vi "Count Objects Reduced.vi"(4 "State In":T1, 6 "Settings":T4={"Objects"=0, "Threshold"=128, "Reject Border"=FALSE, "Fill Holes"=FALSE, "Min Object Size"=FALSE, "Min Size"=3, "Max Object Size"=FALSE, "Max Size"=100, "Show Search Area"=FALSE, "Show Center"=TRUE, "Show Bounding Box"=TRUE} {"Objects" items=["Bright Objects", "Dark Objects"]; "Threshold" min=1 max=999999999 step=1; "Max Size" min=1 max=999999999 step=1; "Min Size" min=1 max=999999999 step=1}, 7 "Low/Tiny":bool, 8 "error in":errorcluster, 9 "Rectangle":T3 {"Rotation" min=-90.0 max=90.0 step=1.0 format="%.2f"; "Left" scale=0.0..1024.0; "Right" scale=0.0..1024.0}, 10 "Temp":T2, 11 "Image":T2) -> (0 "error out":errorcluster, 2 "Objects":T5[](array[typedef]) {"Aspect Ratio" format="%.2f"; "Orientation" format="%.2f"; "Area" format="%.2f"; "Object Center"."Y" format="%.2f"; "Object Center"."X" format="%.2f"}, 3 "Elapsed time (ms)":u32, 5 "Number of Objects":i32)   [LabVIEW 2015]
uses:
  TypeDefs Host/Object Info.ctl
  <vilib>/vision/Image Controls.llb/IMAQ Image.ctl
  TypeDefs Host/States.ctl
  <vilib>/vision/NI_Vision_Development_Module.lvlib
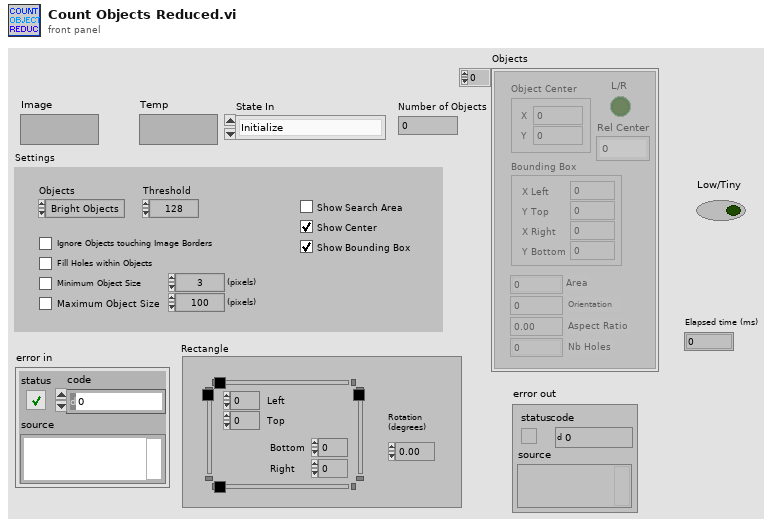
[diagram p1: front panel]
types:
  T1 = typedef "States.ctl" = enum16{"Initialize", "Calibrate", "Create", "Settings", "Shutdown"}
  T2 = typedef "IMAQ Image.ctl" = refnum<image>
  T3 = typedef "IMAQ Rectangle" = cluster{"Left":i32, "Top":i32, "Right":i32, "Bottom":i32, "Rotation":dbl}
  T4 = cluster{"Objects":u16, "Threshold":i32, "Reject Border":bool, "Fill Holes":bool, "Min Object Size":bool, "Min Size":i32, "Max Object Size":bool, "Max Size":i32, "Show Search Area":bool, "Show Center":bool, "Show Bounding Box":bool}
  T5 = typedef "Object Info.ctl" = cluster{"Object Center":cluster{"X":u16, "Y":u16}, "Bounding Box":cluster{"X Left":u16, "Y Top":u16, "X Right":u16, "Y Bottom":u16}, "Area":u16, "Orientation":u16, "Aspect Ratio":sgl, "Nb Holes":u16, "L/R":bool, "Rel Center":u16}
  T6 = typedef "Particle Parameters" = i32
  T7 = cluster{"Measurement Parameter":T6, "Range Lower Value":dbl, "Range Upper Value":dbl, "Range":bool, "Measurement Type":bool}[]
  T8 = typedef "ROI Descriptor" = cluster{"Global Rectangle":i32[], "Contours":cluster{"ID":enum32{"External", "Internal"}, "Type":u32, "Coordinates":i32[]}[]}
  T9 = cluster{"Measurement Parameter":T6, "Range Lower Value":dbl, "Range Upper Value":dbl, "Range":bool, "Measurement Type":bool}
  T10 = cluster{"Global Rectangle[0]":i32, "Global Rectangle[1]":i32}
  T11 = cluster{"[0]":u16, "[1]":u16, "[2]":u16, "[3]":u16, "[4]":u16, "[5]":u16, "[6]":u16, "[7]":u16, "[8]":u16, "[9]":u16, "[10]":u16}
  T12 = cluster{"[2]":u16, "[3]":u16, "[4]":u16, "[5]":u16}
  T13 = cluster{"X Left":u16, "Y Top":u16, "X Right":u16, "Y Bottom":u16}
  T14 = cluster{"Object Center":cluster{"X":u16, "Y":u16}, "Bounding Box":cluster{"X Left":u16, "Y Top":u16, "X Right":u16, "Y Bottom":u16}, "Area":u16, "Orientation":u16, "Aspect Ratio":sgl, "Nb Holes":u16}
  T15 = cluster{"Show Search Area":bool, "Show Center":bool, "Show Bounding Box":bool}
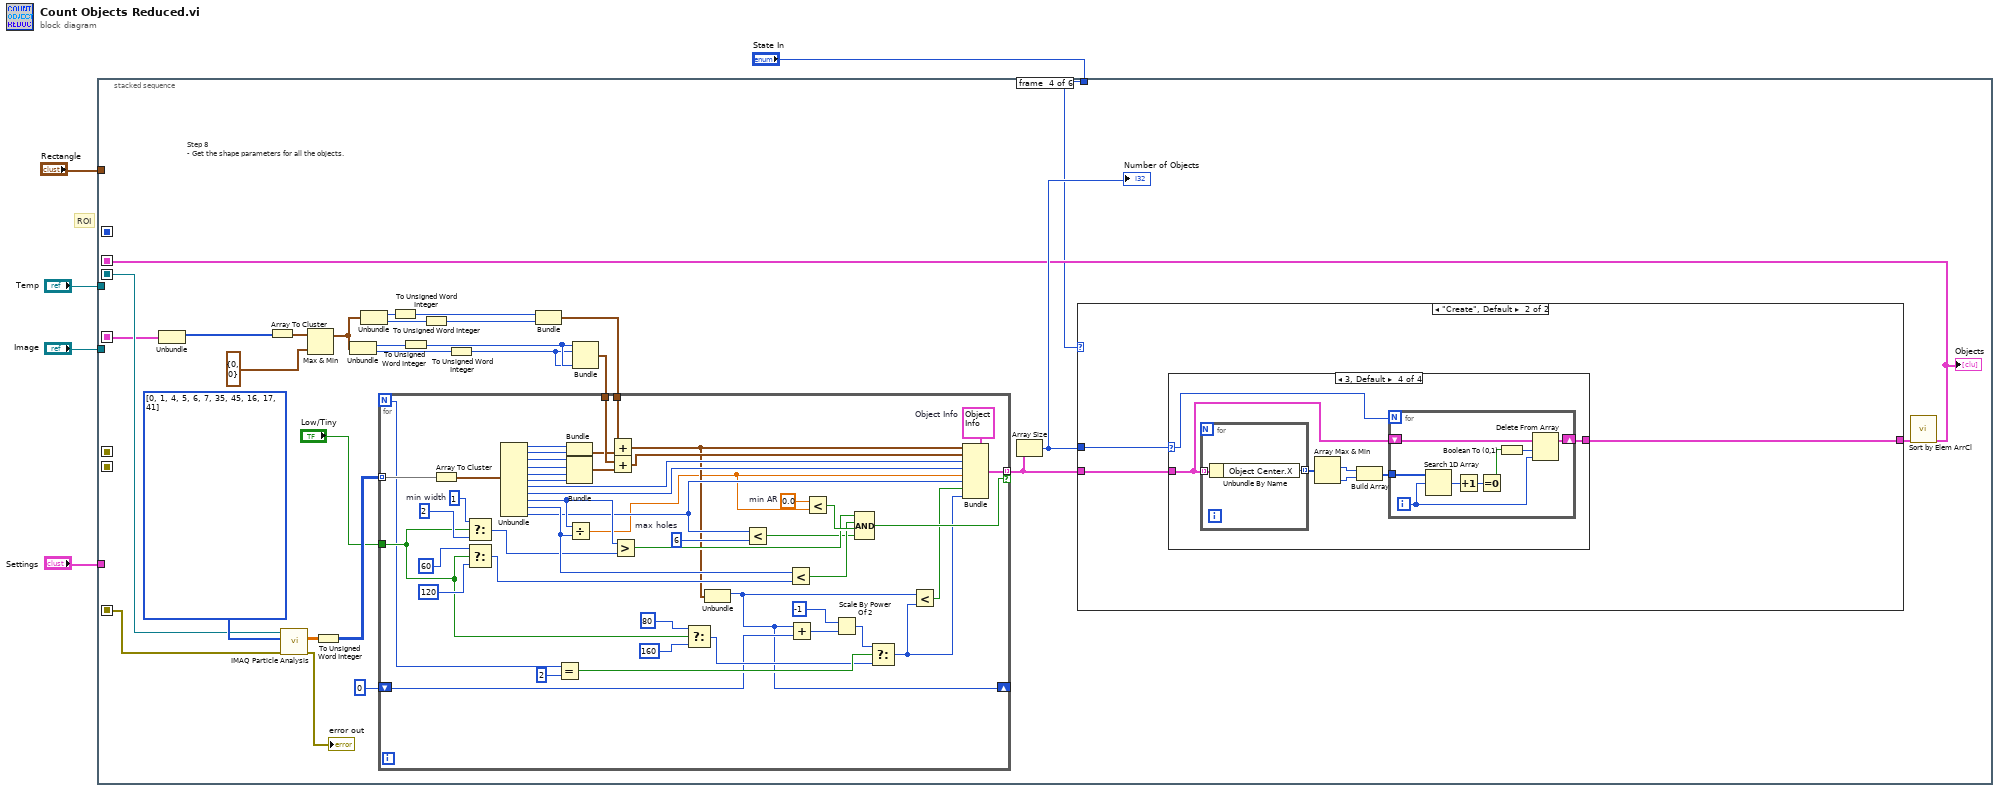
[diagram p0: block diagram]
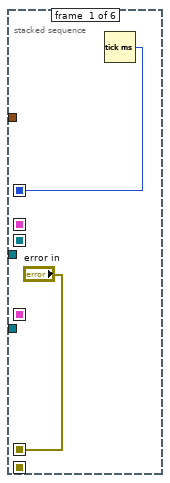
[diagram p2: hidden frame]
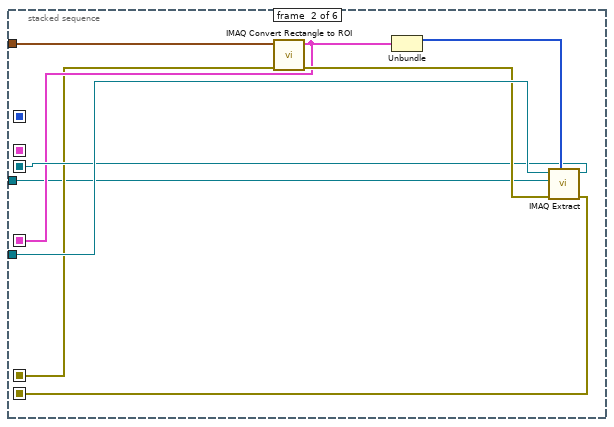
[diagram p3: hidden frame]
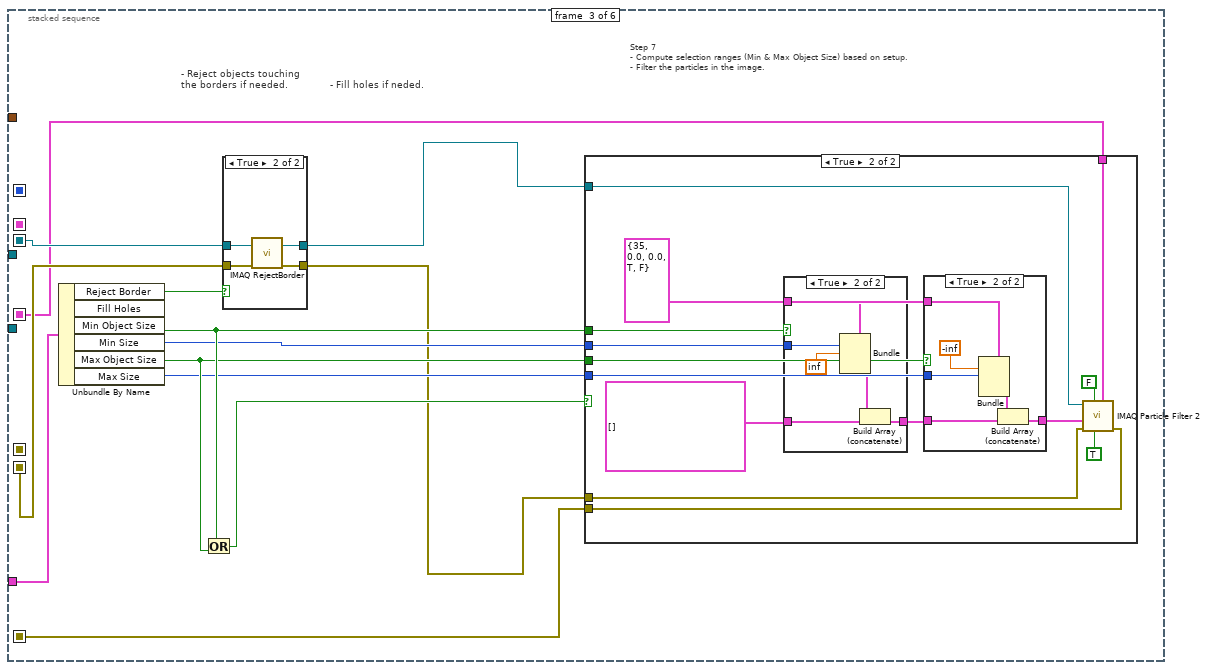
[diagram p4: hidden frame]
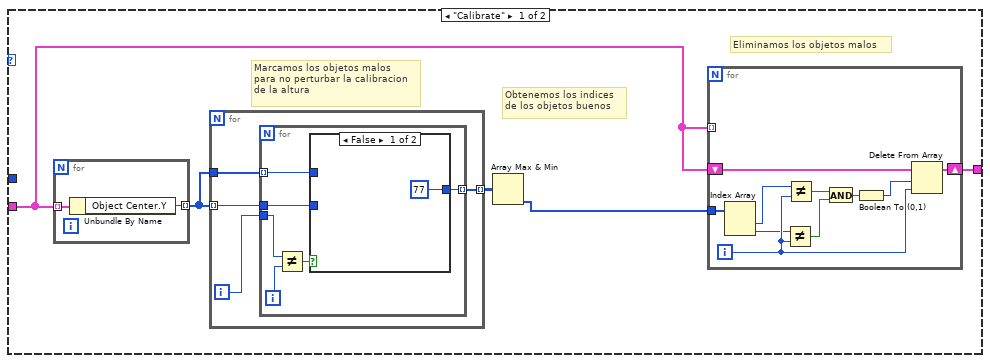
[diagram p9: hidden frame]
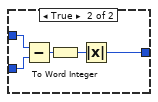
[diagram p10: hidden frame]
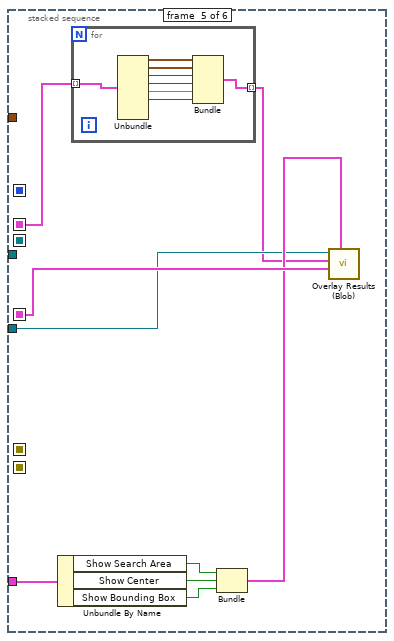
[diagram p14: hidden frame]
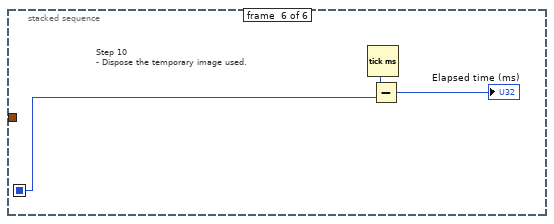
[diagram p15: hidden frame]
diagram:
  # "ROI"
  n1 = stacked-sequence {
    seq-local: [w7 _ _ _ _ _] -> [_ _ _ _ _ w217]
    seq-local: [_ _ _ w67 _ _] -> [_ _ _ _ w202 _]
    seq-local: [_ _ w23 _ _ _] -> [_ _ _ w82 _ _]
    seq-local: ["error in" _ _ _ _ _] -> [_ w9 _ _ _ _]
    seq-local: [_ w12 _ _ _ _] -> [_ _ w22 _ _ _]
    seq-local: [_ w11 _ _ _ _] -> [_ _ w21 w86 _ _]
    seq-local: [_ w10 _ _ _ _] -> [_ _ w19 w85 w201 _]
    tunnel: "Settings" -> [_ _ w28 _ w206 _]
    tunnel: "Image" -> [_ w16 _ _ w199 _]
    tunnel: "Rectangle" -> [_ w14 _ _ _ _]
    tunnel: "Temp" -> [_ w8 _ _ _ _]
    tunnel: "State In" -> [_ _ _ w66 _ _]
    frame #0 {
      n2 = Tick Count (ms)() -> (millisecond timer value=w7:u32)
    }
    frame #1 {
      n3 = call "IMAQ Convert Rectangle to ROI"("error in (no error)"=w9, "Rectangle"=w14) -> ("error out"=w13:errorcluster, "ROI Descriptor"=w10:T8)  [unwired: 7 out]
      n4 = Unbundle(w10) -> ("Global Rectangle"=w15:i32[])  [unwired: 1 out]
      n5 = call "IMAQ Extract"("Optional Rectangle"=w15, "error in (no error)"=w13, "Image Dst"=w8, "Image Src"=w16) -> ("error out"=w12:errorcluster, "Image Dst Out"=w11:T2)  [unwired: 2 in, 4 out]
    }
    frame #2 {
      # "- Fill holes if neded."
      # "- Reject objects touching the borders if needed."
      # "Step 7\n- Compute selection ranges (Min & Max Object Size) based on setup.\n- Filter the particles in the image."
      n6 = Unbundle By Name(w28) -> ("Reject Border"=w20:bool, "Min Object Size"=w27:bool, "Min Size"=w26:i32, "Max Object Size"=w25:bool, "Max Size"=w24:i32)  [unwired: 1 out]
      n7 = Or(x=w27, y=w25) -> (x .or. y?=w29:bool)
      n8 = case shown="True" w20 {
        tunnel: w21 -> [w31 w35]
        tunnel: w22 -> [w30 w34]
        tunnel: [w30 w32] -> w17
        tunnel: [w31 w33] -> w18
        frame False {
        }
        frame True {
          n9 = call "IMAQ RejectBorder"("error in (no error)"=w34, "Image Src"=w35) -> ("error out"=w32:errorcluster, "Image Dst Out"=w33:T2)  [unwired: 2 in, 2 out]
        }
      }
      n10 = case shown="True" w29 {
        tunnel: w27 -> [_ w50]
        tunnel: w26 -> [_ w49]
        tunnel: w25 -> [_ w48]
        tunnel: w24 -> [_ w47]
        tunnel: w17 -> [w36 w45]
        tunnel: [w36 w44] -> w23
        tunnel: w18 -> [_ w38]
        tunnel: w19 -> [_ w37]
        frame False {
        }
        frame True {
          w42 = T9 {"Measurement Parameter"=35, "Range Lower Value"=0.0, "Range Upper Value"=0.0, "Range"=TRUE, "Measurement Type"=FALSE} ("Selection Value")
          n11 = case shown="True" w50 {
            tunnel: T7 [] ("Selection Values") -> [w58 w64]
            tunnel: w49 -> [_ w61]
            tunnel: [w58 w62] -> w40
            tunnel: w42 -> [_ w59]
            frame False {
            }
            frame True {
              n12 = Bundle(cluster=w59, "Range Lower Value"=w61, "Range Upper Value"=inf) -> (w63:T9)  [unwired: 3 out]
              n13 = Build Array (concatenate)(w63, w64) -> (w62:T7)
            }
          }
          n14 = case shown="True" w48 {
            tunnel: w40 -> [w51 w57]
            tunnel: w47 -> [_ w54]
            tunnel: [w51 w55] -> w41
            tunnel: w42 -> [_ w52]
            frame False {
            }
            frame True {
              n15 = Bundle(cluster=w52, "Range Lower Value"=-inf, "Range Upper Value"=w54) -> (w56:T9)  [unwired: 3 out]
              n16 = Build Array (concatenate)(w56, w57) -> (w55:T7)
            }
          }
          n17 = call "IMAQ Particle Filter 2"("ROI Descriptor"=w37, "Keep/Remove Particles (F)"=TRUE ("Keep/Remove Particles"), "Connectivity 4/8 (8)"=FALSE ("Keep/Remove Particles"), "error in (no error)"=w45, "Selection Values"=w41, "Image Src"=w38) -> ("error out"=w44:errorcluster)  [unwired: 2 in, 3 out]
        }
      }
    }
    frame #3 {
      w87 = T6[] [0, 1, 4, 5, 6, 7, 35, 45, 16, 17, 41] items=["Center of Mass X", "Center of Mass Y", "First Pixel X", "First Pixel Y", "Bounding Rect Left", "Bounding Rect Top", "Bounding Rect Right", "Bounding Rect Bottom", "Max Feret Diameter Start X", "Max Feret Diameter Start Y", "Max Feret Diameter End X", "Max Feret Diameter End Y", "Max Horiz. Segment Length Left", "Max Horiz. Segment Length Right", "Max Horiz. Segment Length Row", "-", "Bounding Rect Width", "Bounding Rect Height", "Bounding Rect Diagonal", "Perimeter", "Convex Hull Perimeter", "Holes' Perimeter", "Max Feret Diameter", "Equivalent Ellipse Major Axis", "Equivalent Ellipse Minor Axis", "Equivalent Ellipse Minor Axis (Feret)", "Equivalent Rect Long Side", "Equivalent Rect Short Side", "Equivalent Rect Diagonal", "Equivalent Rect Short Side (Feret)", "Average Horiz. Segment Length", "Average Vert. Segment Length", "Hydraulic Radius", "Waddel Disk Diameter", "-", "Area", "Holes' Area", "Particle & Holes' Area", "Convex Hull Area", "Image Area", "-", "Number of Holes", "Number of Horiz. Segments", "Number of Vert. Segments", "-", "Orientation", "Max Feret Diameter Orientation", "-", "% Area/Image Area", "% Area/(Particle & Holes' Area)", "Ratio of Equivalent Ellipse Axes", "Ratio of Equivalent Rect Sides", "-", "Elongation Factor", "Compactness Factor", "Heywood Circularity Factor", "Type Factor", "-", "Sum X", "Sum Y", "Sum XX", "Sum XY", "Sum YY", "Sum XXX", "Sum XXY", "Sum XYY", "Sum YYY", "-", "Moment of Inertia XX", "Moment of Inertia XY", "Moment of Inertia YY", "Moment of Inertia XXX", "Moment of Inertia XXY", "Moment of Inertia XYY", "Moment of Inertia YYY", "Norm. Moment of Inertia XX", "Norm. Moment of Inertia XY", "Norm. Moment of Inertia YY", "Norm. Moment of Inertia XXX", "Norm. Moment of Inertia XXY", "Norm. Moment of Inertia XYY", "Norm. Moment of Inertia YYY", "Hu Moment 1", "Hu Moment 2", "Hu Moment 3", "Hu Moment 4", "Hu Moment 5", "Hu Moment 6", "Hu Moment 7"] ("Pixel Measurements")
      # "Step 8\n- Get the shape parameters for all the objects."
      n18 = Unbundle(w85) -> ("Global Rectangle"=w84:i32[])  [unwired: 1 out]
      n19 = Array To Cluster(array=w84) -> (cluster=w83:T10)
      n20 = call "IMAQ Particle Analysis"("error in (no error)"=w82, "Pixel Measurements"=w87, "Image"=w86) -> ("error out"=→"error out":errorcluster, "Particle Measurements (Pixels)"=w81:dbl[][])  [unwired: 2 in, 5 out]
      n21 = Max & Min(x=w83, y=cluster{i32, i32} {0, 0}) -> (max(x,y)=w91:cluster{i32, i32})  [unwired: 1 out]
      n22 = To Unsigned Word Integer(number=w81) -> (unsigned 16bit integer=w80:u16[][])
      n23 = Unbundle(w91) -> (w89:i32, w88:i32)
      n24 = Unbundle(w91) -> (w77:i32, w75:i32)
      n25 = To Unsigned Word Integer(number=w77) -> (unsigned 16bit integer=w76:u16)
      n26 = To Unsigned Word Integer(number=w89) -> (unsigned 16bit integer=w79:u16)
      n27 = To Unsigned Word Integer(number=w75) -> (unsigned 16bit integer=w74:u16)
      n28 = To Unsigned Word Integer(number=w88) -> (unsigned 16bit integer=w78:u16)
      n29 = Bundle(w76, w74) -> (w73:cluster{u16, u16})  [unwired: 1 out]
      n30 = Bundle(w79, w78, w79, w78) -> (w90:cluster{u16, u16, u16, u16})  [unwired: 1 out]
      n31 = for {
        N -> [w152]
        tunnel: w80 -> [w187] mode=indexing
        tunnel: w73 -> [w197]
        tunnel: w90 -> [w196]
        tunnel: [w159] -> w71 mode=indexing if=w181
        tunnel: "Low/Tiny" -> [w162]
        shift-right: [w150] -> _
        shift-left: u16 0 ("y") -> [w151]
        w167 = u16 6  # max holes
        w174 = u16 1  # min width
        w180 = sgl 0.0  # min AR
        w186 = T5 {"Object Center"={"X"=0, "Y"=0}, "Bounding Box"={"X Left"=0, "Y Top"=0, "X Right"=0, "Y Bottom"=0}, "Area"=0, "Orientation"=0, "Aspect Ratio"=0.0, "Nb Holes"=0, "L/R"=FALSE, "Rel Center"=0}  # Object Info
        n32 = Array To Cluster(array=w187) -> (cluster=w195:T11)
        n33 = Select(t=w174, s=w162, f=u16 2 ("y")) -> (s? t:f=w169:u16)
        n34 = Select(t=u16 60 ("y"), s=w162, f=u16 120 ("y")) -> (s? t:f=w170:u16)
        n35 = Unbundle(w195) -> ("[0]"=w184:u16, "[1]"=w194:u16, "[2]"=w192:u16, "[3]"=w191:u16, "[4]"=w190:u16, "[5]"=w189:u16, "[6]"=w182:u16, "[7]"=w185:u16, "[8]"=w178:u16, "[9]"=w177:u16, "[10]"=w168:u16)
        n36 = Equal?(x=w152, y=2) -> (x = y?=w164:bool)
        n37 = Bundle("[0]"=w184, "[1]"=w194) -> (w193:cluster{"[0]":u16, "[1]":u16})  [unwired: 1 out]
        n38 = Bundle("[2]"=w192, "[3]"=w191, "[4]"=w190, "[5]"=w189) -> (w188:T12)  [unwired: 1 out]
        n39 = Divide(x=w178, y=w177) -> (x/y=w149:sgl)
        n40 = Add(x=w197, y=w193) -> (x+y=w158:cluster{u16, u16})
        n41 = Add(x=w196, y=w188) -> (x+y=w183:cluster{u16, u16, u16, u16})
        n42 = Greater?(x=w178, y=w169) -> (0:w176:bool)
        n43 = Select(t=u16 80 ("y"), s=w162, f=u16 160) -> (s? t:f=w160:u16)
        n44 = Unbundle(w158) -> (w150:u16)  [unwired: 1 out]
        n45 = Less?(x=w168, y=w167) -> (x < y?=w166:bool)
        n46 = Less?(x=w177, y=w170) -> (x < y?=w175:bool)
        n47 = Add(x=w150, y=w151) -> (x+y=w157:u16)
        n48 = Less?(x=w180, y=w149) -> (x < y?=w179:bool)
        n49 = Scale By Power Of 2(n=i16 -1, x=w157) -> (x*2^n=w155:u16)
        n50 = Compound Arithmetic op=AND(w176, w175, w179, w166) -> (w181:bool)
        n51 = Select(t=w155, s=w164, f=w160) -> (s? t:f=w154:u16)
        n52 = Less?(x=w150, y=w154) -> (x < y?=w153:bool)
        n53 = Bundle(cluster=w186, "Object Center"=w158, "Bounding Box"=w183, "Area"=w182, "Orientation"=w185, "Aspect Ratio"=w149, "Nb Holes"=w168, "L/R"=w153, "Rel Center"=w154) -> (w159:T5)
      }
      n54 = Array Size(array=w71) -> (size(s)=w70:i32)
      "Number of Objects" <- w70
      n55 = case shown="\"Create\", Default" w66 {
        tunnel: w71 -> [w95 w128]
        tunnel: w70 -> [_ w127]
        tunnel: [w96 w126] -> w68
        frame "Calibrate" {
          # "Eliminamos los objetos malos"
          # "Marcamos los objetos malos\npara no perturbar la calibracion\nde la altura"
          # "Obtenemos los indices\nde los objetos buenos"
          n56 = for {
            tunnel: w95 -> [w125] mode=indexing
            tunnel: [w124] -> w97 mode=indexing
            n57 = Unbundle By Name(w125) -> ("Object Center.Y"=w124:u16)
          }
          n58 = for {
            tunnel: w97 -> [w110] mode=indexing
            tunnel: w97 -> [w109]
            tunnel: [w108] -> w94 mode=indexing
            i -> [w111]
            n59 = for {
              tunnel: w111 -> [w116]
              tunnel: w110 -> [w115]
              tunnel: w109 -> [w114] mode=indexing
              tunnel: [w112] -> w108 mode=indexing
              i -> [w113]
              n60 = Not Equal?(x=w116, y=w113) -> (x != y?=w117:bool)
              n61 = case shown="False" w117 {
                tunnel: w115 -> [_ w123]
                tunnel: w114 -> [_ w122]
                tunnel: [i16 77 w119] -> w112
                frame False {
                }
                frame True {
                  n62 = Subtract(x=w122, y=w123) -> (x-y=w121:u16)
                  n63 = To Word Integer(number=w121) -> (16bit integer=w120:i16)
                  n64 = Absolute Value(x=w120) -> (abs(x)=w119:i16)
                }
              }
            }
          }
          n65 = Array Max & Min(array=w94) -> (min index (indices)=w93:i32[])  [unwired: 3 out]
          n66 = for {
            shift-right: [w106] -> w96
            shift-left: w95 -> [w107]
            tunnel: w95 -> [_] mode=indexing
            tunnel: w93 -> [w100]
            i -> [w101]
            n67 = Index Array(array=w100) -> (element #1=w99:i32, element #2=w98:i32)  [unwired: 2 in]
            n68 = Not Equal?(x=w98, y=w101) -> (x != y?=w102:bool)
            n69 = Not Equal?(x=w99, y=w101) -> (x != y?=w103:bool)
            n70 = And(x=w103, y=w102) -> (x .and. y?=w104:bool)
            n71 = Boolean To (0,1)(Boolean=w104) -> (0, 1=w105:i16)
            n72 = Delete From Array(array=w107, length=w105, index=w101) -> (array with subset deleted=w106:T5[])  [unwired: 1 out]
          }
        }
        frame "Create", Default {
          n73 = case shown="3, Default" w127 {
            selector: w127 -> [_ _ _ w132]
            tunnel: w128 -> [w129 w130 w131 w137]
            tunnel: [w129 w130 w131 w138] -> w126
            frame 0 {
            }
            frame 1 {
            }
            frame 2 {
            }
            frame 3, Default {
              n74 = for {
                tunnel: w137 -> [w148] mode=indexing
                tunnel: [w147] -> w136 mode=indexing
                n75 = Unbundle By Name(w148) -> ("Object Center.X"=w147:u16)
              }
              n76 = Array Max & Min(array=w136) -> (max index (indices)=w135:i32, min index (indices)=w134:i32)  [unwired: 2 out]
              n77 = Build Array(w135, w134) -> (w133:i32[])
              n78 = for {
                N: w132 -> [_]
                shift-right: [w145] -> w138
                shift-left: w137 -> [w146]
                tunnel: w133 -> [w144]
                i -> [w139]
                n79 = Search 1D Array(1D array=w144, element=w139) -> (index of element=w143:i32)  [unwired: 1 in]
                n80 = Increment(x=w143) -> (x+1=w142:i32)
                n81 = Equal To 0?(x=w142) -> (x = 0?=w141:bool)
                n82 = Boolean To (0,1)(Boolean=w141) -> (0, 1=w140:i16)
                n83 = Delete From Array(array=w146, length=w140, index=w139) -> (array with subset deleted=w145:T5[])  [unwired: 1 out]
              }
            }
          }
        }
      }
      n84 = call "Sort by Elem ArrCl.vi"("Objects In"=w68) -> ("Objects Out"=w67:T5[])  [unwired: 10 in]
      "Objects" <- w67
    }
    frame #4 {
      n85 = Unbundle By Name(w206) -> ("Show Search Area"=w205:bool, "Show Center"=w204:bool, "Show Bounding Box"=w203:bool)
      n86 = for {
        tunnel: w202 -> [w214] mode=indexing
        tunnel: [w208] -> w198 mode=indexing
        n87 = Unbundle(w214) -> ("Object Center"=w207:cluster{"X":u16, "Y":u16}, "Bounding Box"=w213:T13, "Area"=w212:u16, "Orientation"=w211:u16, "Aspect Ratio"=w210:sgl, "Nb Holes"=w209:u16)  [unwired: 2 out]
        n88 = Bundle("Object Center"=w207, "Bounding Box"=w213, "Area"=w212, "Orientation"=w211, "Aspect Ratio"=w210, "Nb Holes"=w209) -> (w208:T14)  [unwired: 1 in]
      }
      n89 = Bundle("Show Search Area"=w205, "Show Center"=w204, "Show Bounding Box"=w203) -> (w200:T15)  [unwired: 1 out]
      n90 = call <vilib>:"Overlay Results (Blob).vi"("Setup"=w200, "ROI"=w201, "Objects"=w198, "Image In"=w199) -> ()  [unwired: 1 in, 7 out]
    }
    frame #5 {
      # "Step 10\n- Dispose the temporary image used."
      n91 = Tick Count (ms)() -> (millisecond timer value=w216:u32)
      n92 = Subtract(x=w216, y=w217) -> (x-y=→"Elapsed time (ms)":u32)
    }
  }
